vi "Deep Search Priv.vi"(0 "Tree Dictionary In":variant, 5 "Name":string, 11 "error in":errorcluster) -> (4 "Tree Dictionary Out":variant, 6 "IDs":string[](array[string]), 15 "error out":errorcluster)   [LabVIEW 2017, in "Tree API.lvlib" / "Tree.lvclass"]
uses:
  Tree.lvclass
  Typedefs/Tree Cluster.ctl
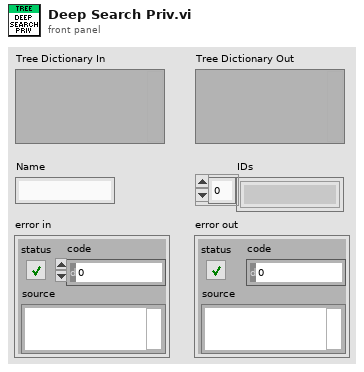
[diagram p1: front panel]
types:
  T1 = typedef "Tree API.lvlib/Tree.lvclass/Tree Cluster.ctl" = cluster{"Unique ID":string, "Parent ID":string, "Child IDs":string[], "Name":string, "MetaData":string, "Data IDs":string[]}
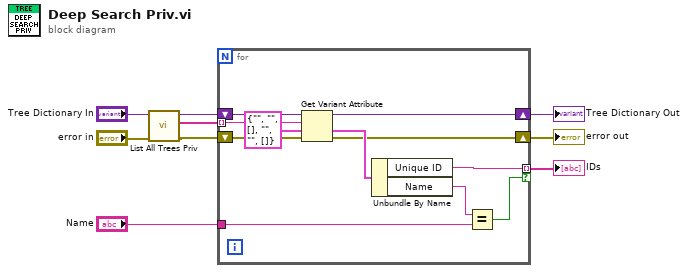
[diagram p0: block diagram]
diagram:
  n1 = call "List All Trees Priv.vi"("error in"="error in", "Tree Dict"="Tree Dictionary In") -> ("error out"=w1:errorcluster, "Tree IDs"=w2:string[], "Tree Dict"=w4:variant)  [unwired: 6 in, 1 out]
  n2 = for {
    tunnel: "Name" -> [w18]
    shift-right: [w14] -> w6
    shift-left: w4 -> [w20]
    tunnel: [w13] -> w8 mode=indexing if=w12
    shift-right: [w15] -> w7
    shift-left: w1 -> [w16]
    tunnel: w2 -> [w11] mode=indexing
    n3 = Get Variant Attribute(Variant=w20, name=w11, default value (empty Variant)=T1 {"Unique ID"="", "Parent ID"="", "Child IDs"=[], "Name"="", "MetaData"="", "Data IDs"=[]} ("Cluster of class private data"), error in=w16) -> (duplicate Variant=w14:variant, value=w19:T1, error out=w15:errorcluster)  [unwired: 1 out]
    n4 = Unbundle By Name(w19) -> ("Unique ID"=w13:string, "Name"=w17:string)
    n5 = Equal?(x=w17, y=w18) -> (x = y?=w12:bool)
  }
  "IDs" <- w8
  "error out" <- w7
  "Tree Dictionary Out" <- w6
